vi "Detect Hardware.vi"(8 "error in (no error)":errorcluster, 11 "Microscope_RM21 in":refnum<class "Microscope_RM21.lvclass">) -> (0 "error out":errorcluster, 3 "Microscope_RM21 out":refnum<class "Microscope_RM21.lvclass">)   [LabVIEW 2020]
uses:
  Microscope_RM21.lvclass
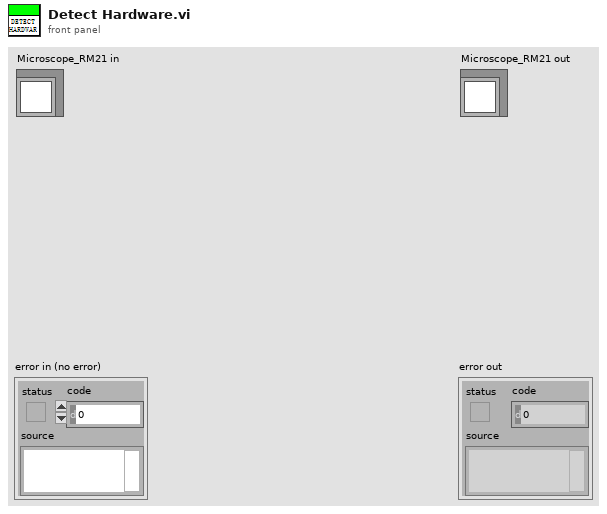
[diagram p1: front panel]
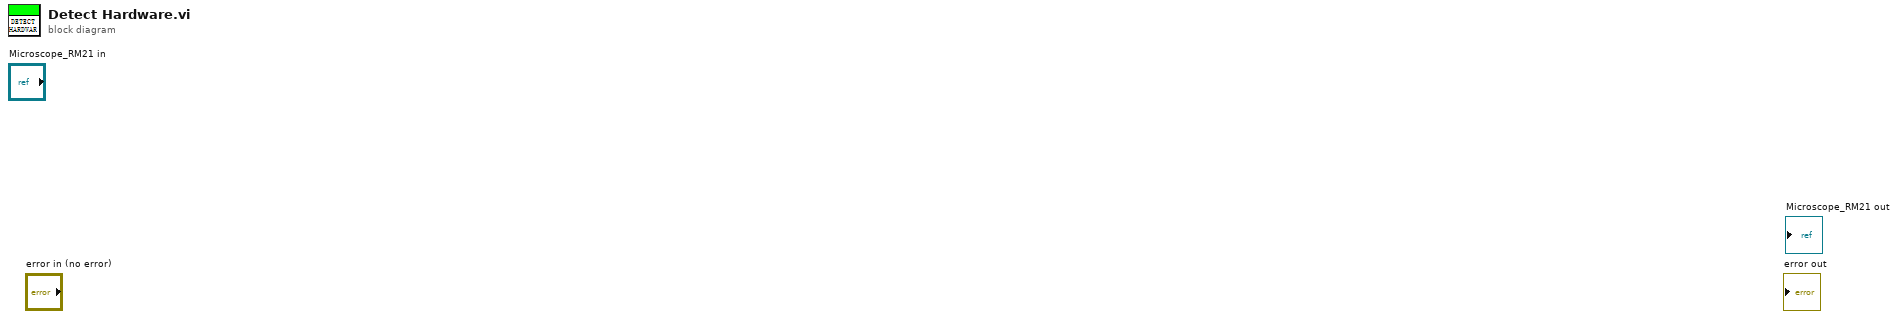
[diagram p0: block diagram]
diagram:
